vi "Process.vi"(8 "error in (no error)":errorcluster, 11 "Coverage Analyzer In":refnum<class "Coverage Analyzer Process.lvclass">) -> (0 "error out":errorcluster, 3 "Coverage Analyzer Out":refnum<class "Coverage Analyzer Process.lvclass">)   [LabVIEW 2020, in "Coverage Analyzer Process.lvclass"]
uses:
  Coverage Analyzer Process.lvclass
  C:/Git/astemes-lunit/source/Application Framework/Process Classes/Process/Process.lvclass
  Application Framework/Process Classes/Process/Process.lvclass/Process.ctl
  Coverage Analyzer Process.lvclass/Coverage Analyzer Process.ctl
  <vilib>/Utility/error.llb/Error Cluster From Error Code.vi
  <vilib>/ErrorRing/Error Ring.xnode
  Application Framework/Process Classes/Process/Process.lvclass
  Coverage Analyzer/Coverage Analyzer.lvclass
  Result Classes/Test Suite Result/Test Suite Result.lvclass
  Result Classes/Test Case Result/Test Case Result.lvclass
  Result Classes/Method Result/Method Result.lvclass
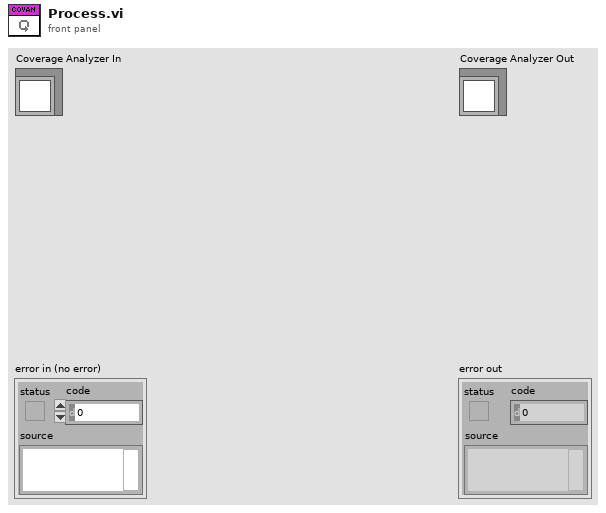
[diagram p1: front panel]
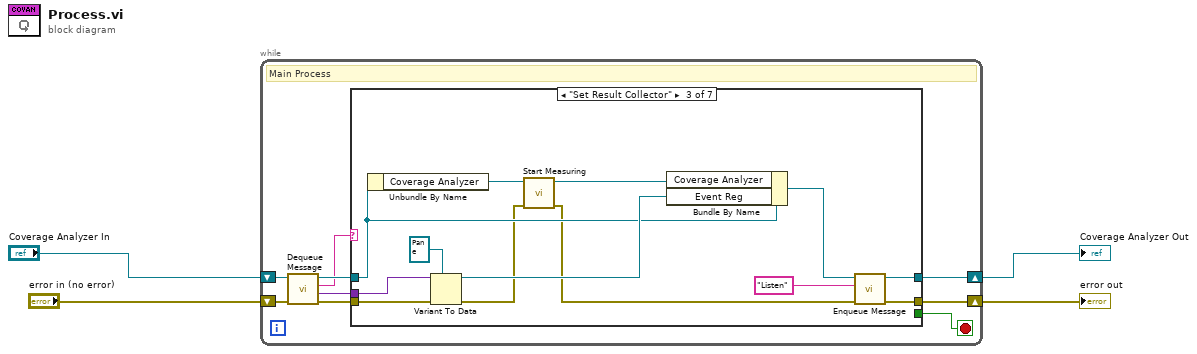
[diagram p0: block diagram]
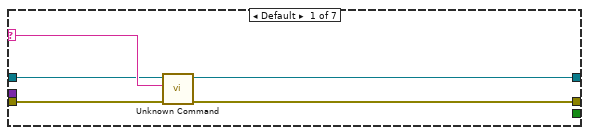
[diagram p2: hidden frame]
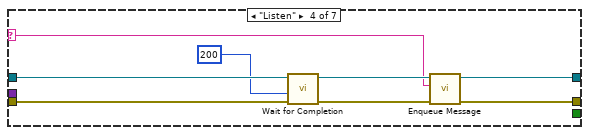
[diagram p4: hidden frame]
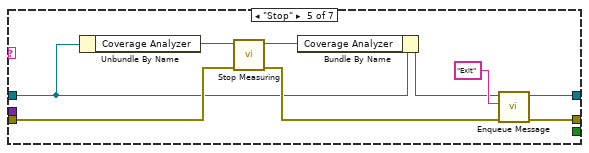
[diagram p5: hidden frame]
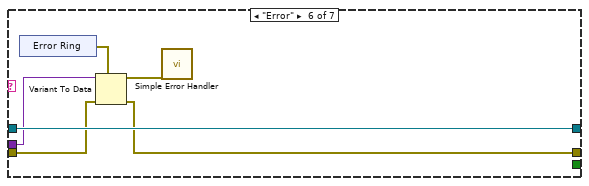
[diagram p6: hidden frame]
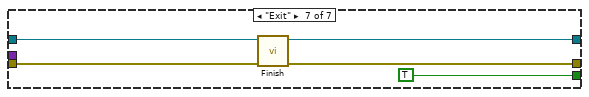
[diagram p7: hidden frame]
diagram:
  n1 = while {
    shift-right: [w8] -> w4
    shift-left: "error in (no error)" -> [w12]
    shift-right: [w10] -> w3
    shift-left: "Coverage Analyzer In" -> [w13]
    stop <- w5 stop-if-true
    # "Main Process"
    n2 = call "Dequeue Message.vi"("error in (no error)"=w12, "Process In"=w13) -> ("error out"=w11:errorcluster, "Message Data"=w6:variant, "Message"=w7:string, "Process Out"=w9:refnum<class "Coverage Analyzer Process.lvclass">)  [unwired: 6 in]
    n3 = case shown="\"Set Result Collector\"" w7 {
      selector: w7 -> [w18 _ _ w35 _ _ _]
      tunnel: [w15 w19 w24 w38 w49 w52 w59] -> w8
      tunnel: w11 -> [w14 w19 w33 w40 w46 w55 w58]
      tunnel: [w17 w20 w27 w36 w48 w56 w60] -> w10
      tunnel: w9 -> [w16 w20 w26 w41 w44 w56 w61]
      tunnel: w6 -> [_ _ w32 _ _ w54 _]
      tunnel: [_ _ _ _ _ _ TRUE] -> w5
      frame Default {
        n4 = call "Unknown Command.vi"("error in (no error)"=w14, "String"=w18, "Process In"=w16) -> ("error out"=w15:errorcluster, "Process Out"=w17:refnum<class "Coverage Analyzer Process.lvclass">)  [unwired: 7 in]
      }
      frame "Init" {
      }
      frame "Set Result Collector" {
        n5 = Unbundle By Name(w26) -> ("Coverage Analyzer"=w25:refnum<class "Coverage Analyzer.lvclass">)
        n6 = Variant To Data(error in=w33, type=refnum<event-registration> refnum ("Event Registration Refnum"), Variant=w32) -> (data=w30:refnum<event-registration>, error out=w22:errorcluster)
        n7 = call "Start Measuring.vi"("error in (no error)"=w22, "Coverage Analyzer in"=w25) -> ("error out"=w21:errorcluster, "Coverage Analyzer out"=w23:refnum<class "Coverage Analyzer.lvclass">)  [unwired: 8 in]
        n8 = Bundle By Name(cluster=w26, "Coverage Analyzer"=w23, "Event Reg"=w30) -> (w29:refnum<class "Coverage Analyzer Process.lvclass">)
        n9 = call "Enqueue Message.vi"("error in (no error)"=w21, "Message"="Listen", "Process In"=w29) -> ("error out"=w24:errorcluster, "Process Out"=w27:refnum<class "Coverage Analyzer Process.lvclass">)  [unwired: 7 in]
      }
      frame "Listen" {
        n10 = call "Wait for Completion.vi"("error in (no error)"=w40, "Timeout"=200, "Coverage Analyzer Process in"=w41) -> ("error out"=w39:errorcluster, "Coverage Analyzer Process out"=w37:refnum<class "Coverage Analyzer Process.lvclass">)  [unwired: 7 in]
        n11 = call "Enqueue Message.vi"("error in (no error)"=w39, "Message"=w35, "Process In"=w37) -> ("error out"=w38:errorcluster, "Process Out"=w36:refnum<class "Coverage Analyzer Process.lvclass">)  [unwired: 7 in]
      }
      frame "Stop" {
        n12 = Unbundle By Name(w44) -> ("Coverage Analyzer"=w43:refnum<class "Coverage Analyzer.lvclass">)
        n13 = call "Stop Measuring.vi"("error in (no error)"=w46, "Coverage Analyzer in"=w43) -> ("error out"=w47:errorcluster, "Coverage Analyzer out"=w42:refnum<class "Coverage Analyzer.lvclass">)  [unwired: 8 in]
        n14 = Bundle By Name(cluster=w44, "Coverage Analyzer"=w42) -> (w45:refnum<class "Coverage Analyzer Process.lvclass">)
        n15 = call "Enqueue Message.vi"("error in (no error)"=w47, "Message"="Exit", "Process In"=w45) -> ("error out"=w49:errorcluster, "Process Out"=w48:refnum<class "Coverage Analyzer Process.lvclass">)  [unwired: 7 in]
      }
      frame "Error" {
        n16 = xnode "Error Ring"() -> ("error out"=w53:errorcluster)
        n17 = Variant To Data(error in=w55, type=w53, Variant=w54) -> (data=w51:errorcluster, error out=w52:errorcluster)
        n18 = call <vilib>:"Simple Error Handler.vi"("error in (no error)"=w51) -> ()  [unwired: 4 in, 5 out]
      }
      frame "Exit" {
        n19 = call "Finish.vi"("error in (no error)"=w58, "Process In"=w61) -> ("error out"=w59:errorcluster, "Process Out"=w60:refnum<class "Coverage Analyzer Process.lvclass">)  [unwired: 8 in]
      }
    }
  }
  "error out" <- w4
  "Coverage Analyzer Out" <- w3
